vi "numeric to cDAQ thread id enum.vi"(11 "Numeric":i32) -> (3 "Station cDAQ Thread Queues out":T1=enum."tcp comms")   [LabVIEW 2012]
uses:
  typedefs/station cDAQ thread IDs.ctl
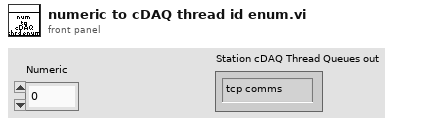
[diagram p1: front panel]
types:
  T1 = typedef "station cDAQ thread IDs.ctl" = enum16{"cDAQ main", "analog input", "eol test exe", "nvh test exe", "tcp comms"}
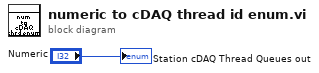
[diagram p0: block diagram]
diagram:
  "Station cDAQ Thread Queues out" <- "Numeric"
